vi "ALTS-2015 DB Write Result Driver.vi"(7 "Operation":T2, 8 "Error In":errorcluster, 11 "DB Write Result Options":T1) -> (0 "error out":errorcluster)   [LabVIEW 2013]
doc: "Copyright © 2005, Soliton Technologies.\nAll rights reserved."
uses:
  <vilib>/addons/database/Auxilliary.llb/DB Tools Parameter Info.ctl
  <vilib>/addons/database/Auxilliary.llb/DB Tools DataTypes.ctl
  <vilib>/addons/database/Auxilliary.llb/DB Tools Parameter Dir.ctl
  Controls/ALTS-2015 Write DB Write Result Driver Cases.ctl
  Controls/ALTS-2015 write DB Result cases.ctl
  Controls/ALTS-2015 LV2GBL Options.ctl
  <vilib>/addons/database/Command.llb/Cmd ObjectReference.ctl
  <vilib>/addons/database/Connection.llb/DB Tools Open Connec (Path).vi
  <vilib>/addons/database/Command.llb/Cmd Delete.vi
  <vilib>/addons/database/NI_Database_API.lvlib
panel:
  out "Time (ms)":u32
  out "parameters out":T3[](array[typedef])
  out "DB Procedure- Write Result":string
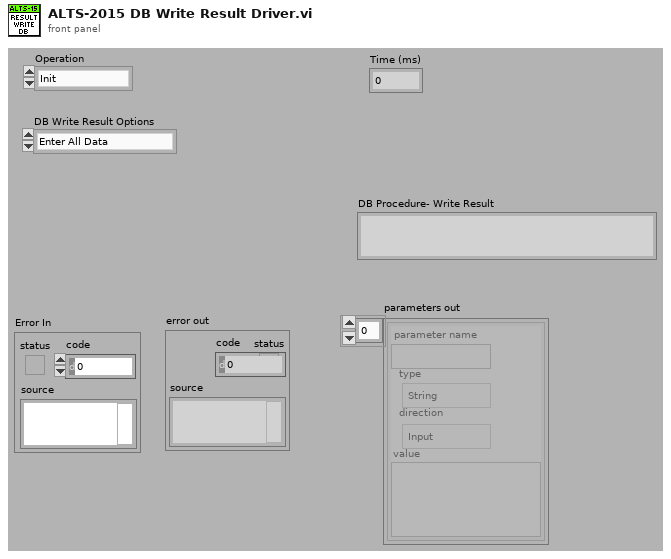
[diagram p1: front panel]
types:
  T1 = typedef "ALTS-2015 write DB Result cases.ctl" = enum16{"Enter All Data", "Enter WO & SN"}
  T2 = typedef "ALTS-2015 Write DB Write Result Driver Cases.ctl" = enum16{"Init", "Write Result", "Close"}
  T3 = typedef "NI_Database_API.lvlib/DB Tools Parameter Info.ctl" = cluster{"parameter name":string, "type":T4, "direction":T5, "value":variant}
  T4 = typedef "NI_Database_API.lvlib/DB Tools DataTypes.ctl" = enum16{"String", "Long (I32)", "Single (SGL)", "Double (DBL)", "Date/Time", "Binary"}
  T5 = typedef "NI_Database_API.lvlib/DB Tools Parameter Dir.ctl" = enum32{"Input", "Output", "Input/Output", "Return Value"}
  T6 = typedef "ALTS-2015 LV2GBL Options.ctl" = enum16{"Read all", "Write all"}
  T7 = typedef "ALTS-2015 INI Configuration Cluster.ctl" = cluster{"Application":cluster{"Rerun Count":i32, "Workorder No":string}, "Station Details":cluster{"Sensor Name 1":string, "Sensor Name 2":string, "Sensor Name 3":string, "Sensor Name 4":string, "Station1 Enable":bool, "Station2 Enable":bool, "Station3 Enable":bool, "Station4 Enable":bool}, "Database":cluster{"Database Connection Link":path, "Result Procedure":string, "User":string, "Password":string, "Prompt":bool, "Station 1 LT Result DB DSN Path":path, "Station 2 LT Result DB DSN Path":path, "Station 3 LT Result DB DSN Path":path, "Station 4 LT Result DB DSN Path":path, "AirLeakTestResult Procedure":string, "Serial Details Procedure":string}, "Simulation":cluster{"Simulate DAQ Hardware":bool, "Simulate Result DB Write":bool, "Simulate Scanner":bool, "Simulate OPC":bool, "Simulate Serial Details DB":bool, "Simulate Result DB":bool, "Simulate Scanner DB Path":path, "Simulate Serial Details DB Path":path, "Simulate Result DB Path":path}, "Barcode Scanner1":cluster{"Scanner IP":string, "Scanner Port":u16, "#Bytes to Read":i32}, "Barcode Scanner2":cluster{"Enabled?":bool, "Scanner IP":string, "Scanner Port":u16, "#Bytes to Read":i32}}
  T8 = typedef "NI_Database_API.lvlib/Conn ObjectReference.ctl" = refnum<k1>
  T9 = typedef "NI_Database_API.lvlib/Cmd ObjectReference.ctl" = refnum<k1>
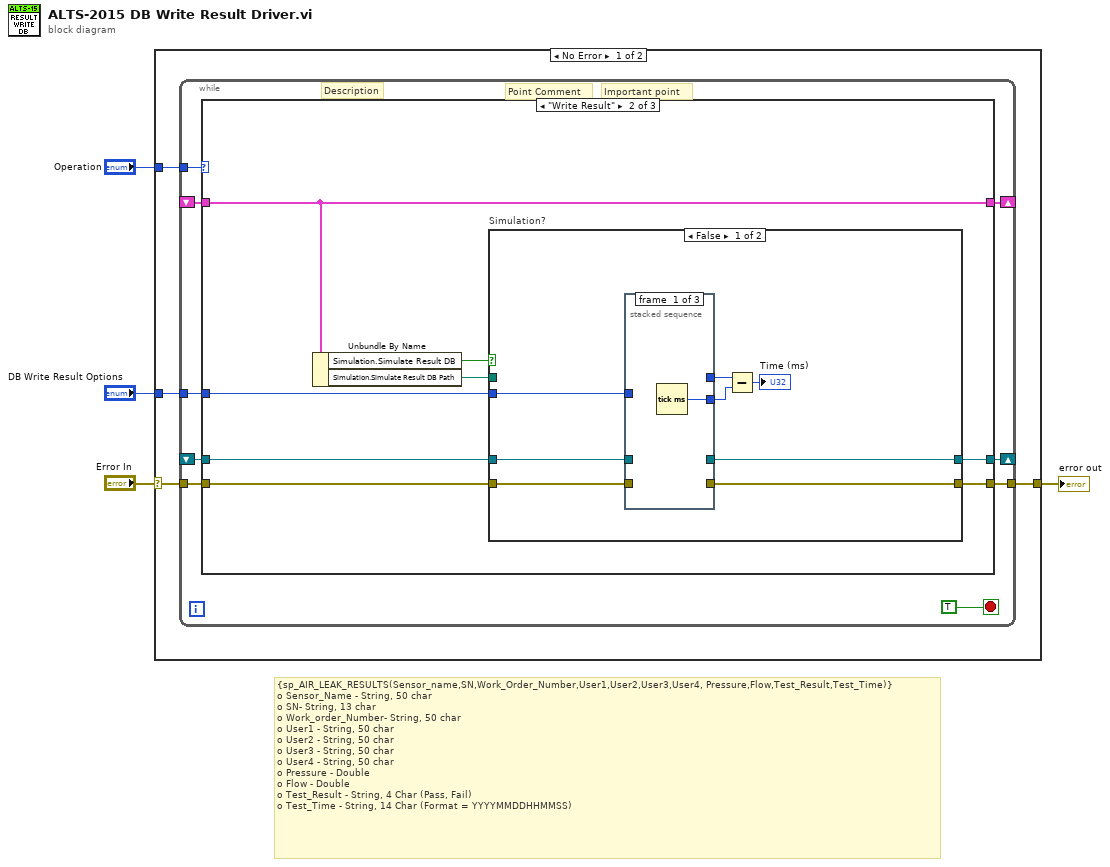
[diagram p0: block diagram]
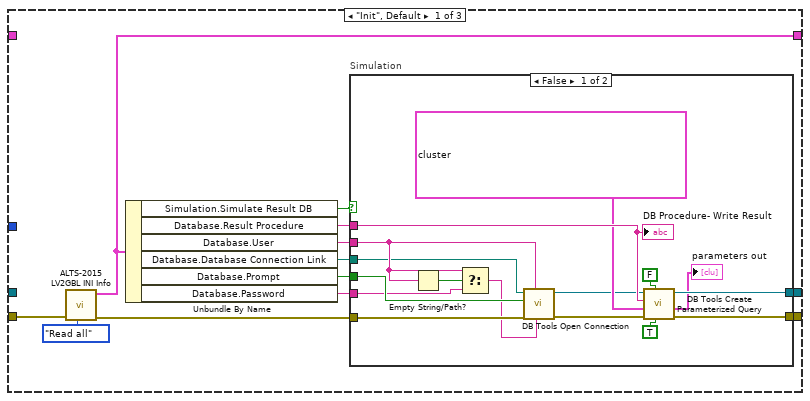
[diagram p2: hidden frame]
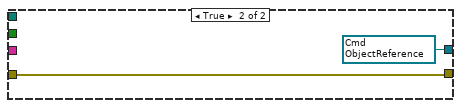
[diagram p3: hidden frame]
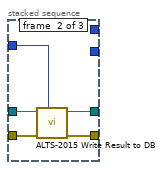
[diagram p4: hidden frame]
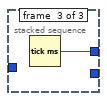
[diagram p5: hidden frame]
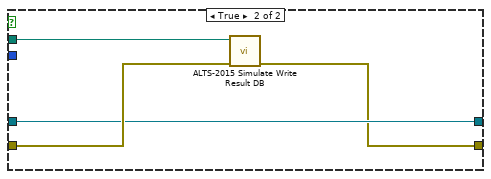
[diagram p6: hidden frame]
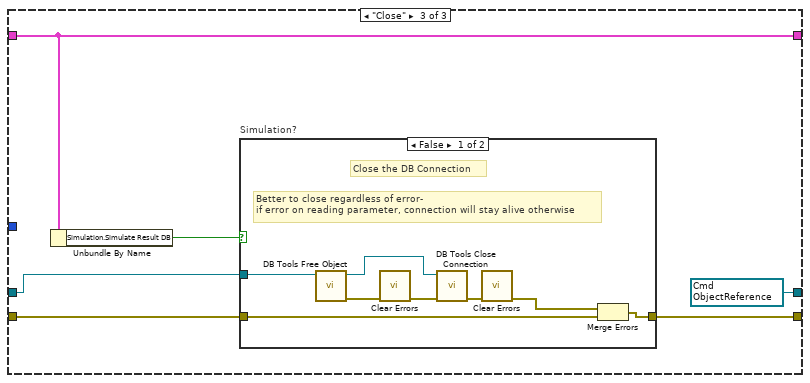
[diagram p7: hidden frame]
diagram:
  # "{sp_AIR_LEAK_RESULTS(Sensor_name,SN,Work_Order_Number,User1,User2,User3,User4, Pressure,Flow,Test_Result,Test_Time)}\no\tSensor_Name - String, 50 char\no\tSN- String, 13 char\no\tWork_order_Number- String, 50 char\no\tUser1 - String, 50 char\no\tUser2 - String, 50 char\no\tUser3 - String, 50 char\no\tUser4 - String, 50 char\no\tPressure - Double\no\tFlow - Double\no\tTest_Result - String, 4 Char (Pass, Fail)\no\tTest_Time - String, 14 Char (Format = YYYYMMDDHHMMSS)"
  n1 = case shown="No Error" "Error In" {
    selector: "Error In" -> [w7 w90]
    tunnel: [w8 w90] -> w4
    tunnel: "Operation" -> [w6 _]
    tunnel: "DB Write Result Options" -> [w5 _]
    frame No Error {
      # "Point Comment"
      # "Important point"
      # "Description"
      n2 = while {
        tunnel: [w16] -> w8
        shift-right: [w15] -> _
        shift-left: _ -> [w14]
        tunnel: w7 -> [w13]
        tunnel: w6 -> [w12]
        tunnel: w5 -> [w11]
        shift-right: [w10] -> _
        shift-left: _ -> [w9]
        stop <- TRUE stop-if-true
        n3 = case shown="\"Write Result\"" w12 {
          tunnel: w13 -> [w29 w52 w77]
          tunnel: [w23 w53 w80] -> w16
          tunnel: [w24 w54 w78] -> w15
          tunnel: w14 -> [_ w55 w79]
          tunnel: w11 -> [_ w51 _]
          tunnel: [w18 w50 w76] -> w10
          tunnel: w9 -> [_ w50 w76]
          frame "Init", Default {
            n4 = call "ALTS-2015 LV2GBL INI Info.vi"("Options"=ALTS-2015_LV2GBL_Options."Read all", "error in"=w29) -> ("error out"=w28:errorcluster, "Configuration Cluster Out"=w18:T7)  [unwired: 8 in]
            n5 = Unbundle By Name(w18) -> ("Simulation.Simulate Result DB"=w19:bool, "Database.Result Procedure"=w22:string, "Database.User"=w25:string, "Database.Database Connection Link"=w21:path, "Database.Prompt"=w27:bool, "Database.Password"=w26:string)
            n6 = case "Simulation" shown="False" w19 {
              tunnel: w28 -> [w45 w47]
              tunnel: w27 -> [w44 _]
              tunnel: w26 -> [w43 _]
              tunnel: w25 -> [w42 _]
              tunnel: [w41 w46] -> w24
              tunnel: [w40 w47] -> w23
              tunnel: w22 -> [w39 _]
              tunnel: w21 -> [w37 _]
              frame False {
                n7 = Empty String/Path?(string/path=w42) -> (empty?=w36:bool)
                n8 = Select(t=w42, s=w36, f=w43) -> (s? t:f=w35:string)
                n9 = call-poly <vilib>:"DB Tools Open Connection.vi"("password"=w35, "userID"=w42, "error in (no error)"=w45, "prompt? (F)"=w44, "connection information"=w37) -> ("error out"=w31:errorcluster, "connection reference"=w32:T8)  [unwired: 3 in]
                n10 = call <vilib>:"DB Tools Create Parameterized Query.vi"("stored procedure? (F)"=TRUE ("stored procedure? (f)"), "auto-detect parameters? (F)"=FALSE ("auto-detect parameters? (f)"), "error in (no error)"=w31, "parameters"=T3[] [{"parameter name"="Sensor_Name", "type"=enum."String", "direction"=enum."Input", "value"=variant}, {"parameter name"="SN", "type"=enum."String", "direction"=enum."Input", "value"=variant}, {"parameter name"="WO", "type"=enum."String", "direction"=enum."Input", "value"=variant}, {"parameter name"="User1", "type"=enum."String", "direction"=enum."Input", "value"=variant}, {"parameter name"="User2", "type"=enum."String", "direction"=enum."Input", "value"=variant}, {"parameter name"="User3", "type"=enum."String", "direction"=enum."Input", "value"=variant}, {"parameter name"="User4", "type"=enum."String", "direction"=enum."Input", "value"=variant}, {"parameter name"="P", "type"=enum."Double (DBL)", "direction"=enum."Input", "value"=variant}, {"parameter name"="Flow", "type"=enum."Double (DBL)", "direction"=enum."Input", "value"=variant}, {"parameter name"="TestResult", "type"=enum."String", "direction"=enum."Input", "value"=variant}, {"parameter name"="TestTime", "type"=enum."String", "direction"=enum."Input", "value"=variant}], "SQL query"=w39, "connection reference"=w32) -> ("error out"=w40:errorcluster, "parameters out"=→"parameters out":T3[], "command reference"=w41:T9)  [unwired: 1 in]
                "DB Procedure- Write Result" <- w39
              }
              frame True {
                w46 = T9 refnum items=["Command"] ("command reference")
              }
            }
          }
          frame "Write Result" {
            n11 = Unbundle By Name(w50) -> ("Simulation.Simulate Result DB"=w49:bool, "Simulation.Simulate Result DB Path"=w48:path)
            n12 = case "Simulation?" shown="False" w49 {
              tunnel: w55 -> [w63 w73]
              tunnel: [w62 w73] -> w54
              tunnel: [w61 w72] -> w53
              tunnel: w52 -> [w60 w74]
              tunnel: w51 -> [w56 _]
              tunnel: w48 -> [_ w71]
              frame False {
                n13 = stacked-sequence {
                  tunnel: w63 -> [_ w69 _]
                  tunnel: [_ w68 _] -> w62
                  tunnel: [_ w67 _] -> w61
                  tunnel: w60 -> [_ w65 _]
                  tunnel: [_ _ w70] -> w59
                  tunnel: [w64 _ _] -> w58
                  tunnel: w56 -> [_ w66 _]
                  frame #0 {
                    n14 = Tick Count (ms)() -> (millisecond timer value=w64:u32)
                  }
                  frame #1 {
                    n15 = call "ALTS-2015 Write Result to DB.vi"("Options"=w66, "Error In"=w65, "Command reference In"=w69) -> ("Error Out"=w67:errorcluster, "Command reference Out"=w68:T9)  [unwired: 7 in]
                  }
                  frame #2 {
                    n16 = Tick Count (ms)() -> (millisecond timer value=w70:u32)
                  }
                }
                n17 = Subtract(x=w59, y=w58) -> (x-y=→"Time (ms)":u32)
              }
              frame True {
                n18 = call "ALTS-2015 Simulate Write Result DB.vi"("error in"=w74, "Simulate Result DB Path"=w71) -> ("error out"=w72:errorcluster)  [unwired: 9 in]
              }
            }
          }
          frame "Close" {
            w78 = T9 refnum items=["Command"] ("Command reference Out")
            n19 = Unbundle By Name(w76) -> ("Simulation.Simulate Result DB"=w75:bool)
            n20 = case "Simulation?" shown="False" w75 {
              tunnel: [w88 w89] -> w80
              tunnel: w79 -> [w87 _]
              tunnel: w77 -> [w86 w89]
              frame False {
                # "Better to close regardless of error-\nif error on reading parameter, connection will stay alive otherwise"
                # "Close the DB Connection"
                n21 = call-poly <vilib>:"DB Tools Free Object.vi"("command reference"=w87) -> ("error out"=w85:errorcluster, "connection reference"=w83:T8)  [unwired: 9 in]
                n22 = call <vilib>:"Clear Errors.vi"("error in (no error)"=w85) -> ("error out"=w84:errorcluster)  [unwired: 6 in]
                n23 = call <vilib>:"DB Tools Close Connection.vi"("error in (no error)"=w84, "connection reference"=w83) -> ("error out"=w82:errorcluster)  [unwired: 5 in]
                n24 = call <vilib>:"Clear Errors.vi"("error in (no error)"=w82) -> ("error out"=w81:errorcluster)  [unwired: 6 in]
                n25 = Merge Errors(w81, w86) -> (w88:errorcluster)
              }
              frame True {
              }
            }
          }
        }
      }
    }
    frame Error {
    }
  }
  "error out" <- w4
